vi "Lab-4 a.vi"() -> ()   [LabVIEW 2020]
uses:
  GV/Global 2.vi
panel:
  in  "stop 2":bool
  out "abs(x)":dbl
  out "Chart-2":dbl(graph)
  out "Chart-1":dbl(graph)
  in  "stop":bool
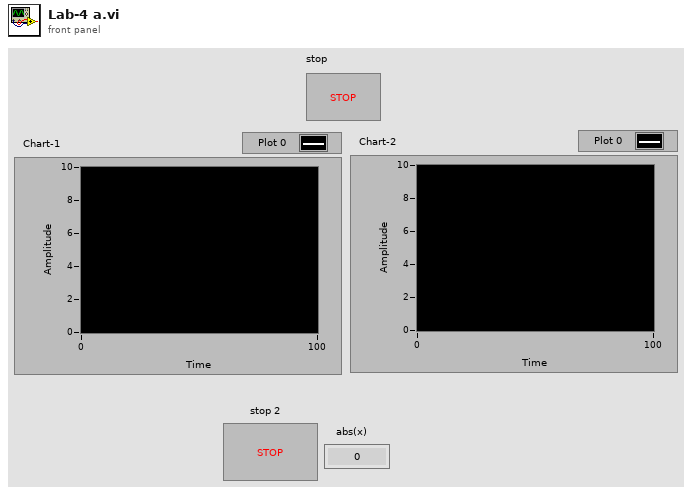
[diagram p1: front panel]
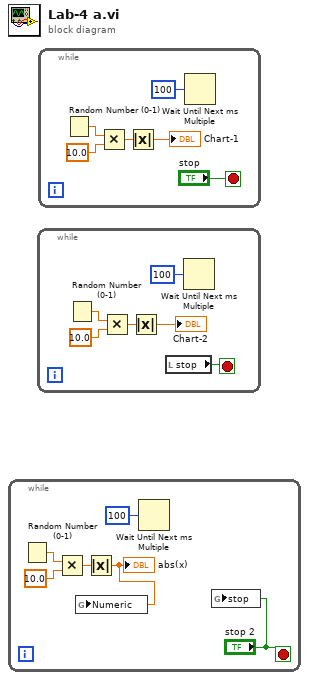
[diagram p0: block diagram]
diagram:
  n1 = while {
    stop <- "stop 2" stop-if-true
    n2 = Random Number (0-1)() -> (number: 0 to 1=w4:dbl)
    n3 = Multiply(x=w4, y=10.0) -> (x*y=w6:dbl)
    n4 = Absolute Value(x=w6) -> (abs(x)=w1:dbl)
    "abs(x)" <- w1
    n5 = global write "Global 2.vi" "Numeric"(w1) -> ()
    n6 = Wait Until Next ms Multiple(millisecond multiple=u32 100) -> ()  [unwired: 1 out]
    n7 = global write "Global 2.vi" "stop"("stop 2") -> ()
  }
  n8 = while {
    stop <- w7 stop-if-true
    n9 = Random Number (0-1)() -> (number: 0 to 1=w10:dbl)
    n10 = Multiply(x=w10, y=10.0) -> (x*y=w12:dbl)
    n11 = Absolute Value(x=w12) -> (abs(x)=→"Chart-2":dbl)
    n12 = local read "stop"() -> (w7:bool)
    n13 = Wait Until Next ms Multiple(millisecond multiple=u32 100) -> ()  [unwired: 1 out]
  }
  n14 = while {
    stop <- "stop" stop-if-true
    n15 = Random Number (0-1)() -> (number: 0 to 1=w18:dbl)
    n16 = Multiply(x=w18, y=10.0) -> (x*y=w16:dbl)
    n17 = Absolute Value(x=w16) -> (abs(x)=→"Chart-1":dbl)
    n18 = Wait Until Next ms Multiple(millisecond multiple=u32 100) -> ()  [unwired: 1 out]
  }
